vi "alphaguesssub.vi"(1 "Input array":dbl[](array[numeric])=[-0.00030713525390624997, -0.00028586572265625, -0.00027093945312499997, -0.00022545166015625, -0.0002288515625, -0.0002832607421875, -0.00026047119140625, -0.00023886328124999998, -0.00024652246093749997, -0.00021825439453124998, -0.00018607080078125, -0.000247435546875, -0.00025890820312499997, -0.000261873046875, -0.00021293164062499999, -0.0002475107421875, -0.000236650390625, -0.00022960888671874998, -0.0002525595703125, -0.00022141796875, -0.00025230712890625, -0.00020463330078125, -0.000219333984375, -0.00022067138671875, -0.0002084521484375, -0.00022530126953124998, -0.000233599609375, -0.0001690712890625, -0.000186849609375, -0.00018957275390625, -0.0002326435546875, -0.0002419140625, -0.0002015126953125, -0.0001390361328125, -0.0001888154296875, -0.00018802050781249998, -0.0002193017578125, -0.00017484521484375, -0.000161927734375, -0.00012102685546875, -0.0001320751953125, -0.00018154296874999998, -0.0001737548828125, -0.000190265625, -0.00017344873046875, -0.00011039208984375, -0.0001356845703125, -0.000154365234375, -0.00023907275390625, -0.000178814453125, -0.00012609179687499998, -0.00010478466796874999, -6.620410156249999e-05, -0.0001212041015625, -0.00012066699218749999, -0.00014433740234375, -0.00013588330078125, -0.00011227734374999999, -4.835595703125e-05, -9.973046874999999e-05, -0.00011135888671875, -0.0001362001953125, -9.2189453125e-05, -6.796582031249999e-05, -7.7236328125e-06, -4.0455078125e-05, -2.362744140625e-05, -7.578076171875e-05, -3.6625488281249996e-05, -2.717236328125e-05, -3.7275390624999996e-05, 8.421875e-06, -6.920654296875e-05, -5.6826171874999995e-06, -6.556494140625e-05, 3.39453125e-06, 1.66396484375e-05, 3.956884765625e-05, 5.47421875e-05, 3.95849609375e-05, 6.11982421875e-05, 3.53525390625e-05, 9.73779296875e-05, 6.905615234375e-05, 3.10126953125e-05, 0.0001309150390625, 8.755419921875e-05, 9.14482421875e-05, 0.0001237392578125, 0.00012848193359375, 0.00014031982421875, 0.00015039599609375, 0.00013820361328125, 0.00018066748046875, 0.000210052734375, 0.00017707421874999999, 0.00021403271484375, 0.00023057568359375, 0.00021669140625, 0.00026155078125, 0.00028294921875, 0.00022386181640625, 0.00026150781249999997, 0.0002730556640625, 0.00029523291015625, 0.00033243310546875, 0.00036490136718749996, 0.00034065087890625, 0.00033635400390624997, 0.0004055927734375, 0.00042370947265625, 0.000407171875, 0.00048352734374999996, 0.000455060546875, 0.0005000810546875, 0.00051623193359375, 0.00048264111328125, 0.00051098974609375, 0.00057723681640625, 0.0005650122070312499, 0.0005770703125, 0.00063009912109375, 0.0006357548828125, 0.00059887158203125, 0.00066485009765625, 0.0006821718749999999, 0.00071149267578125, 0.0006948422851562499, 0.00072468408203125, 0.0007792651367187499, 0.0008093701171875, 0.00081497216796875, 0.00079840771484375, 0.00080429443359375, 0.00082922705078125, 0.00085587841796875, 0.000952703125, 0.0009431640625, 0.0009407470703125, 0.0009460429687499999, 0.00097268359375, 0.00097681396484375, 0.00108295751953125, 0.0010664091796875, 0.00105700439453125, 0.00110888916015625, 0.00109849609375, 0.0011712368164062499, 0.00119464404296875, 0.0012154892578125, 0.00124992333984375, 0.00128349267578125, 0.001293337890625, 0.0012938212890625, 0.00132845947265625, 0.00137615478515625, 0.0013442880859374999, 0.00146242529296875, 0.0014384970703125, 0.0014347265625, 0.00147894677734375, 0.001506806640625, 0.00159572509765625, 0.0015589169921875, 0.00157672216796875, 0.0016231875, 0.00163816748046875, 0.00170148193359375, 0.0017407714843749999, 0.0017298627929687499, 0.001765005859375, 0.0018030869140625, 0.00183484619140625, 0.00188117724609375, 0.0019418115234375, 0.0019461298828125, 0.00196757666015625, 0.0020050185546875, 0.00202544482421875, 0.00203882421875, 0.002112, 0.0021131279296875, 0.00211729052734375, 0.00216484619140625, 0.0022012568359374997, 0.00228121630859375, 0.00229173828125, 0.00226447998046875, 0.00231971630859375, 0.00232337939453125, 0.0024246728515625, 0.00240779150390625, 0.0024507119140625, 0.00248166015625, 0.00246542333984375, 0.0025242099609375, 0.00258820654296875, 0.0025856875, 0.0026379267578125, 0.002646638671875, 0.0026913369140625, 0.0027206953125, 0.00277096875, 0.0027951494140625, 0.002792560546875, 0.00273772705078125, 0.002854134765625, 0.0028010844726562498, 0.00290197509765625, 0.0028956372070312497, 0.00298322900390625, 0.0029761982421875, 0.00300142626953125, 0.0029750434570312498, 0.0030531767578124997, 0.00301610009765625, 0.0031355693359375, 0.0030855375976562498, 0.00312756103515625, 0.00315237548828125, 0.003175412109375, 0.00318658935546875, 0.00321730126953125, 0.00323705078125, 0.00327393408203125, 0.003205103515625, 0.0033012299804687497, 0.0033232568359375, 0.0033226337890625, 0.003367869140625, 0.0033219892578125, 0.0033100009765624997, 0.00338641552734375, 0.00329686865234375, 0.0034094091796875, 0.0034100107421875, 0.00336363134765625, 0.003356912109375, 0.00331527001953125, 0.00334318896484375, 0.0033896328125, 0.00333337060546875, 0.0033256953125, 0.00323339306640625, 0.00330670849609375, 0.0032687509765625, 0.00323555224609375, 0.00327454638671875, 0.00315382568359375, 0.0031024189453124997, 0.00316360107421875, 0.0031080532226562497, 0.00314304052734375, 0.00306474609375, 0.00303264306640625, 0.00306393505859375, 0.00301614306640625, 0.00301225439453125, 0.0029575283203125, 0.00291179345703125, 0.002928900390625, 0.0028338212890625, 0.00284926318359375, 0.002798318359375, 0.0027865771484375, 0.0028124013671875, 0.0027162587890625, 0.00269779296875, 0.00273616943359375, 0.00265690283203125, 0.0026531591796875, 0.0025906074218749998, 0.00261244091796875, 0.002572732421875, 0.00252747021484375, 0.00250374072265625, 0.00255968603515625, 0.0024747314453125, 0.0024555673828125, 0.0024198173828125, 0.0024579790039062498, 0.0023639365234375, 0.0023963564453125, 0.00235060009765625, 0.0022838857421875, 0.00229615869140625, 0.00231847021484375, 0.0022736591796875, 0.00229382763671875, 0.00226535546875, 0.0022270703125, 0.002212611328125, 0.00214448974609375, 0.0021524765625, 0.002117048828125, 0.0020875615234375, 0.00208144384765625, 0.00199998046875, 0.0020216635742187497, 0.0019985087890624998, 0.00199719287109375, 0.00198283056640625, 0.0019428374023437499, 0.00196387060546875, 0.00196988623046875, 0.0018807529296875, 0.0018680341796874999, 0.0018321660156249999, 0.00179855908203125, 0.001800798828125, 0.00175426904296875, 0.0017732880859375, 0.00176222900390625, 0.00170755126953125, 0.0017383115234375, 0.00163319921875, 0.00169230810546875, 0.00159851806640625, 0.00157795751953125, 0.0015402041015625, 0.0014946357421875, 0.00150455078125, 0.00152806005859375, 0.0014818686523437499, 0.001480251953125, 0.00147992431640625, 0.0014072856445312499, 0.00141188330078125, 0.001433609375, 0.0014249619140625, 0.0013497451171875, 0.00133984619140625, 0.00128959423828125, 0.0012686845703124999, 0.00131112158203125, 0.0012658271484374999, 0.00122757421875, 0.00119986474609375, 0.0011720263671874999, 0.001220462890625, 0.0012039736328125, 0.0011738525390625, 0.00115494091796875, 0.0010711518554687499, 0.0010742187499999999, 0.00108722216796875, 0.00103131982421875, 0.00106317041015625, 0.00101475, 0.0010134072265625, 0.0009692890625, 0.000953111328125, 0.00101314404296875, 0.0009563071289062499, 0.0009342587890625, 0.0008854033203124999, 0.0008535634765625, 0.0008618779296875, 0.0008335615234375, 0.0008424077148437499, 0.00085625439453125, 0.000806287109375, 0.0007929399414062499, 0.0008020654296875, 0.0008261494140625, 0.00079469091796875, 0.0007423388671875, 0.0007116376953125, 0.000726365234375, 0.00069750634765625, 0.00072470556640625, 0.00069674365234375, 0.0006323818359375, 0.0006093720703125, 0.00062889599609375, 0.0006252705078125, 0.0005994033203125, 0.00061565625, 0.00059641162109375, 0.00056844970703125, 0.000591529296875, 0.00058839794921875, 0.0005759692382812499, 0.0005574604492187499, 0.0004820126953125, 0.0005025732421875, 0.0004893603515625, 0.00047733984375, 0.0004918095703125, 0.00045772998046875, 0.00045637646484375, 0.00040996484375, 0.0004040029296875, 0.00043732519531249997, 0.00045829931640625, 0.00040354638671875, 0.00037651904296875, 0.0003660185546875, 0.000312576171875, 0.00036642138671875, 0.0003870517578125, 0.0003657607421875, 0.0002723896484375, 0.00028206298828125, 0.00032149755859375, 0.00028822900390625, 0.00031592773437499997, 0.00030765625, 0.00027138525390625, 0.00023873974609375, 0.0002249306640625, 0.00024828955078125, 0.00027435009765625, 0.000258994140625, 0.0001974951171875, 0.00018648974609374998, 0.0001617666015625, 0.00018617822265625, 0.000187, 0.00018515234375, 0.0001203662109375, 0.00010710498046875, 7.857373046875e-05, 0.00013526025390625, 0.000195271484375, 0.00011643994140625, 0.00011173486328124999, 9.45419921875e-05, 7.84072265625e-05, 0.00013478759765625, 0.000140572265625, 0.00010285107421875, 6.0671874999999996e-05, 2.5845703125e-05, 4.520849609375e-05, 5.0901855468749996e-05, 4.803369140625e-05, 6.999609375e-05, 1.15478515625e-06, -3.13671875e-06, -9.66796875e-07, 1.742919921875e-05, 1.4931640625e-06, 7.2509765625e-06, -5.678857421875e-05, -3.7962890625e-05, -5.3469238281249996e-05, -3.4525390625e-05, -2.9986816406249998e-05, -5.70087890625e-05, -9.225390625e-05, -6.630615234375e-05, -9.050830078125e-05, -6.018310546875e-05, -4.497216796875e-05, -6.716552734374999e-05, -0.000109677734375, -9.57880859375e-05, -8.301025390625e-05, -0.0001126533203125, -3.98427734375e-05, -6.63544921875e-05, -8.96435546875e-05, -8.868212890625e-05, -0.00012086572265625, -0.00011960888671874999, -9.305419921875e-05, -0.00015532666015625, -0.00019103369140625, -0.000141904296875, -0.0001810703125, -0.00015786181640625, -0.0001320966796875, -0.000175720703125, -0.0002200537109375, -0.00020896240234375, -0.00021692236328125, -0.00020758740234375, -0.000204466796875, -0.0002208271484375, -0.00018759619140625, -0.00025333837890625, -0.00022699316406249998, -0.00017228857421874998, -0.00017473779296875, -0.000180146484375, -0.0002766435546875, -0.0002868271484375, -0.00023608642578124998, -0.0002178837890625, -0.00021700830078124998, -0.00024114599609375, -0.0002551591796875, -0.00028079541015624997, -0.0002629580078125, -0.00022667089843749998, -0.00023105908203125, -0.00024868701171875, -0.000279103515625, -0.00027006396484375, -0.00027866308593749997, -0.00023139208984375, -0.00024552880859375, -0.00023636572265625, -0.0002849150390625, -0.00031110986328125, -0.00029171484375, -0.00025994482421875, -0.00023096240234375, -0.00025392919921875, -0.00029143017578125, -0.00030062548828125, -0.000292875, -0.0002754189453125, -0.00025728076171875, -0.00028383544921875, -0.00032003125, -0.00034214404296875, -0.00033056396484375, -0.00030305322265625, -0.00028276123046875, -0.0003202568359375, -0.00033010205078125, -0.00034521630859374997, -0.00034471679687499997, -0.00031103466796875, -0.00025710888671875, -0.00032932861328125] format="%.2e") -> (0 "alpha guess":dbl=39.70463667028981 format="%.2f")   [LabVIEW 2013]
panel:
  out "Output Variable":dbl format="%.2f"
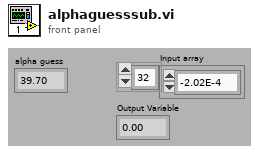
[diagram p1: front panel]
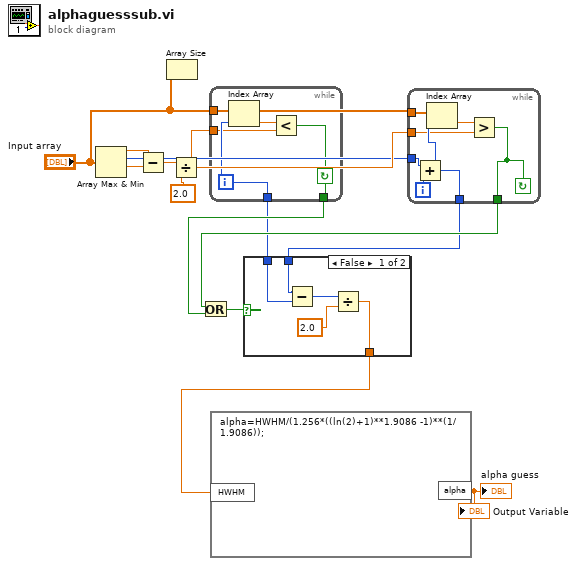
[diagram p0: block diagram]
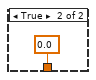
[diagram p2: hidden frame]
diagram:
  n1 = Array Max & Min(array="Input array") -> (max value=w14:dbl, max index (indices)=w4:i32, min value=w13:dbl)  [unwired: 1 out]
  n2 = Subtract(x=w14, y=w13) -> (x-y=w12:dbl)
  n3 = Array Size(array="Input array") -> ()  [unwired: 1 out]
  n4 = Divide(x=w12, y=2.0) -> (x/y=w9:dbl)
  n5 = while {
    tunnel: [w19] -> w5
    tunnel: [w15] -> w7
    tunnel: w9 -> [w17]
    tunnel: "Input array" -> [w18]
    i -> [w19]
    stop <- w15 continue-if-true
    n6 = Index Array(array=w18, index=w19) -> (element=w16:dbl)
    n7 = Less?(x=w16, y=w17) -> (x < y?=w15:bool)
  }
  n8 = while {
    tunnel: [w23] -> w3
    tunnel: w4 -> [w25]
    tunnel: [w20] -> w6
    tunnel: w9 -> [w22]
    tunnel: "Input array" -> [w26]
    i -> [w24]
    stop <- w20 continue-if-true
    n9 = Add(x=w25, y=w24) -> (x+y=w23:i32)
    n10 = Index Array(array=w26, index=w23) -> (element=w21:dbl)
    n11 = Greater?(x=w21, y=w22) -> (0:w20:bool)
  }
  n12 = Or(x=w6, y=w7) -> (x .or. y?=w8:bool)
  n13 = case shown="False" w8 {
    tunnel: w5 -> [w29 _]
    tunnel: w3 -> [w28 _]
    tunnel: [w27 0.0] -> w2
    frame False {
      n14 = Subtract(x=w28, y=w29) -> (x-y=w30:i32)
      n15 = Divide(x=w30, y=2.0) -> (x/y=w27:dbl)
    }
    frame True {
    }
  }
  n16 = formula code="alpha=HWHM/(1.256*((ln(2)+1)**1.9086 -1)**(1/1.9086));"("HWHM"=w2) -> ("alpha"=→"alpha guess" →"Output Variable":dbl)
